vi "Banda_HMI.vi"() -> ()   [LabVIEW 2026]
uses:
  <vilib>/Modbus/master/Create Master Instance (Serial).vi
  <vilib>/Modbus/master/Modbus Master.lvclass
panel:
  in  "stop":bool
  out "Sobrecalentamiento":bool
  out "Contador de piezas":dbl
  out "Temperatura":dbl(slide) scale=0.0..100.0
  out "Sensor de Presencia":bool
  in  "Brazo clasificador":bool
  in  "Velocidad Motor":dbl(knob) scale=0.0..100.0
  in  "Motor ON/OFF":bool
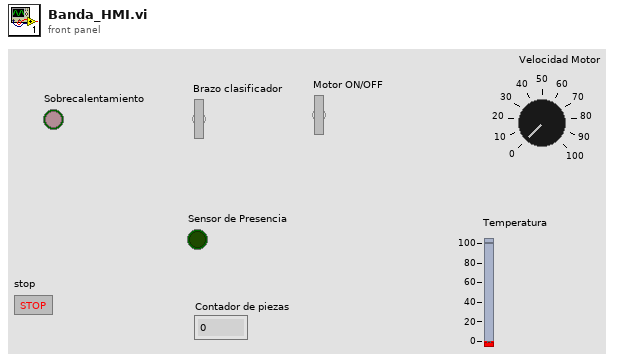
[diagram p1: front panel]
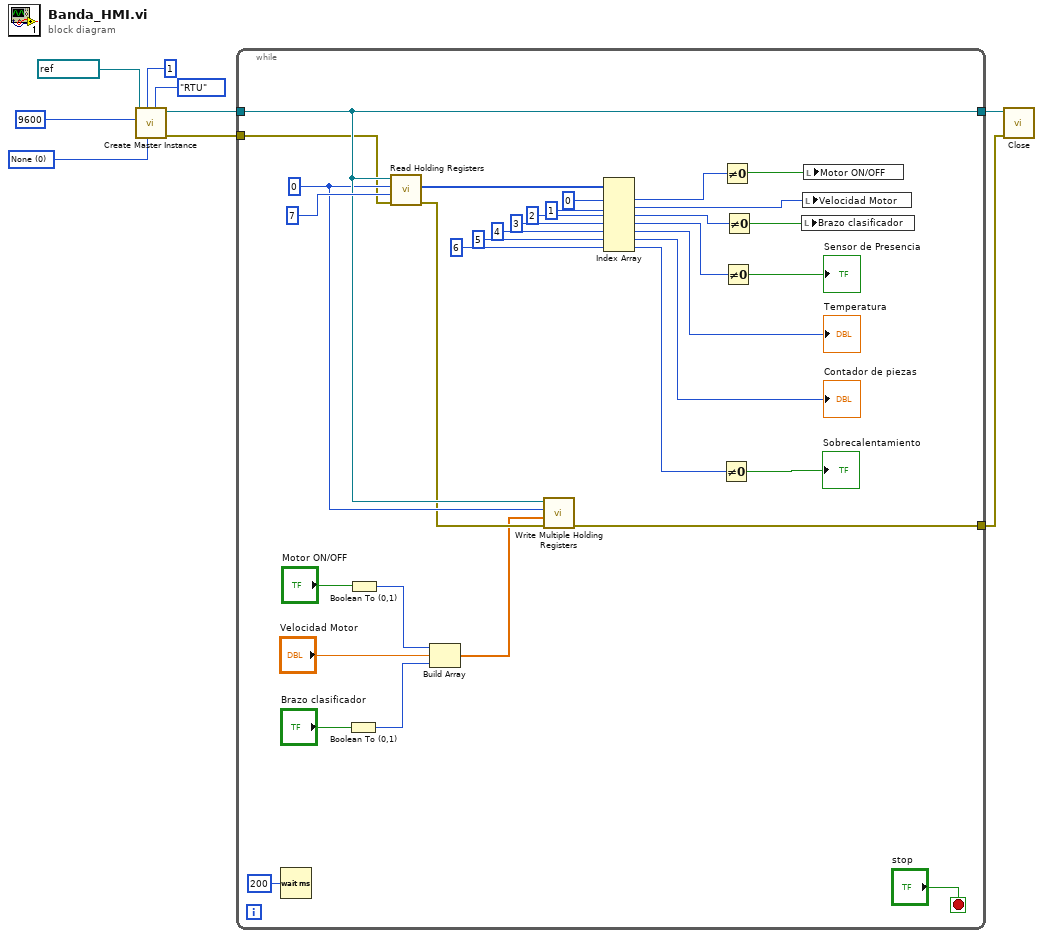
[diagram p0: block diagram]
diagram:
  w5 = u16 0 items=["None", "Odd", "Even"] ("parity (Even)")
  n1 = call-poly <vilib>:"Create Master Instance.vi"("serial type"=enum16{"RTU", "ASCII"}."RTU", "parity (Even)"=w5, "unit ID"=u8 1, "baud rate (9600)"=u32 9600, "VISA resource name"=refnum<visa-resource-name> "COM4") -> ("error out"=w2:errorcluster, "serial master instance"=w9:refnum<class "Modbus Master.lvclass">)  [unwired: 5 in]
  n2 = while {
    tunnel: w9 -> [w20]
    tunnel: [w20] -> w8
    tunnel: w2 -> [w18]
    tunnel: [w10] -> w1
    stop <- "stop" stop-if-true
    w19 = u16 0 ("starting address")
    n3 = Wait (ms)(milliseconds to wait=u32 200) -> ()  [unwired: 1 out]
    n4 = Boolean To (0,1)(Boolean="Brazo clasificador") -> (0, 1=w15:i16)
    n5 = Boolean To (0,1)(Boolean="Motor ON/OFF") -> (0, 1=w12:i16)
    n6 = call-dynamic "Read Holding Registers.vi"("error in (no error)"=w18, "number of holding registers"=u16 7, "starting address"=w19, "Modbus master in"=w20) -> ("error out"=w17:errorcluster, "register values"=w39:u16[])  [unwired: 5 in, 1 out]
    n7 = Build Array(w12, "Velocidad Motor", w15) -> (w11:dbl[])
    n8 = call-dynamic "Write Multiple Holding Registers.vi"("error in (no error)"=w17, "holding register values"=w11, "starting address"=w19, "Modbus master in"=w20) -> ("error out"=w10:errorcluster)  [unwired: 6 in, 1 out]
    n9 = Index Array(array=w39, index #1=0 ("index"), index #2=1 ("index"), index #3=2 ("index"), index #4=3 ("index"), index #5=4 ("index"), index #6=5 ("index"), index #7=6 ("index")) -> (element #1=w31:u16, element #2=w22:u16, element #3=w30:u16, element #4=w29:u16, element #5=→"Temperatura":u16, element #6=→"Contador de piezas":u16, element #7=w26:u16)
    n10 = Not Equal To 0?(x=w26) -> (x != 0?=→"Sobrecalentamiento":bool)
    n11 = Not Equal To 0?(x=w31) -> (x != 0?=w23:bool)
    n12 = Not Equal To 0?(x=w29) -> (x != 0?=→"Sensor de Presencia":bool)
    n13 = Not Equal To 0?(x=w30) -> (x != 0?=w21:bool)
    n14 = local write "Brazo clasificador"(w21) -> ()
    n15 = local write "Velocidad Motor"(w22) -> ()
    n16 = local write "Motor ON/OFF"(w23) -> ()
  }
  n17 = call-dynamic "Close.vi"("error in (no error)"=w1, "Modbus master in"=w8) -> ()  [unwired: 9 in, 1 out]
